vi "Indexing_Modbus.vi"(0 "Modbus master in":refnum<class "Modbus Master.lvclass">, 4 "Modbus Input":T1, 7 "error in (no error)":errorcluster) -> (20 "Modbus master out":refnum<class "Modbus Master.lvclass">, 27 "error out":errorcluster)   [LabVIEW 2021]
uses:
  <vilib>/Modbus/master/Modbus Master.lvclass
  Controls/Modbus Input.ctl
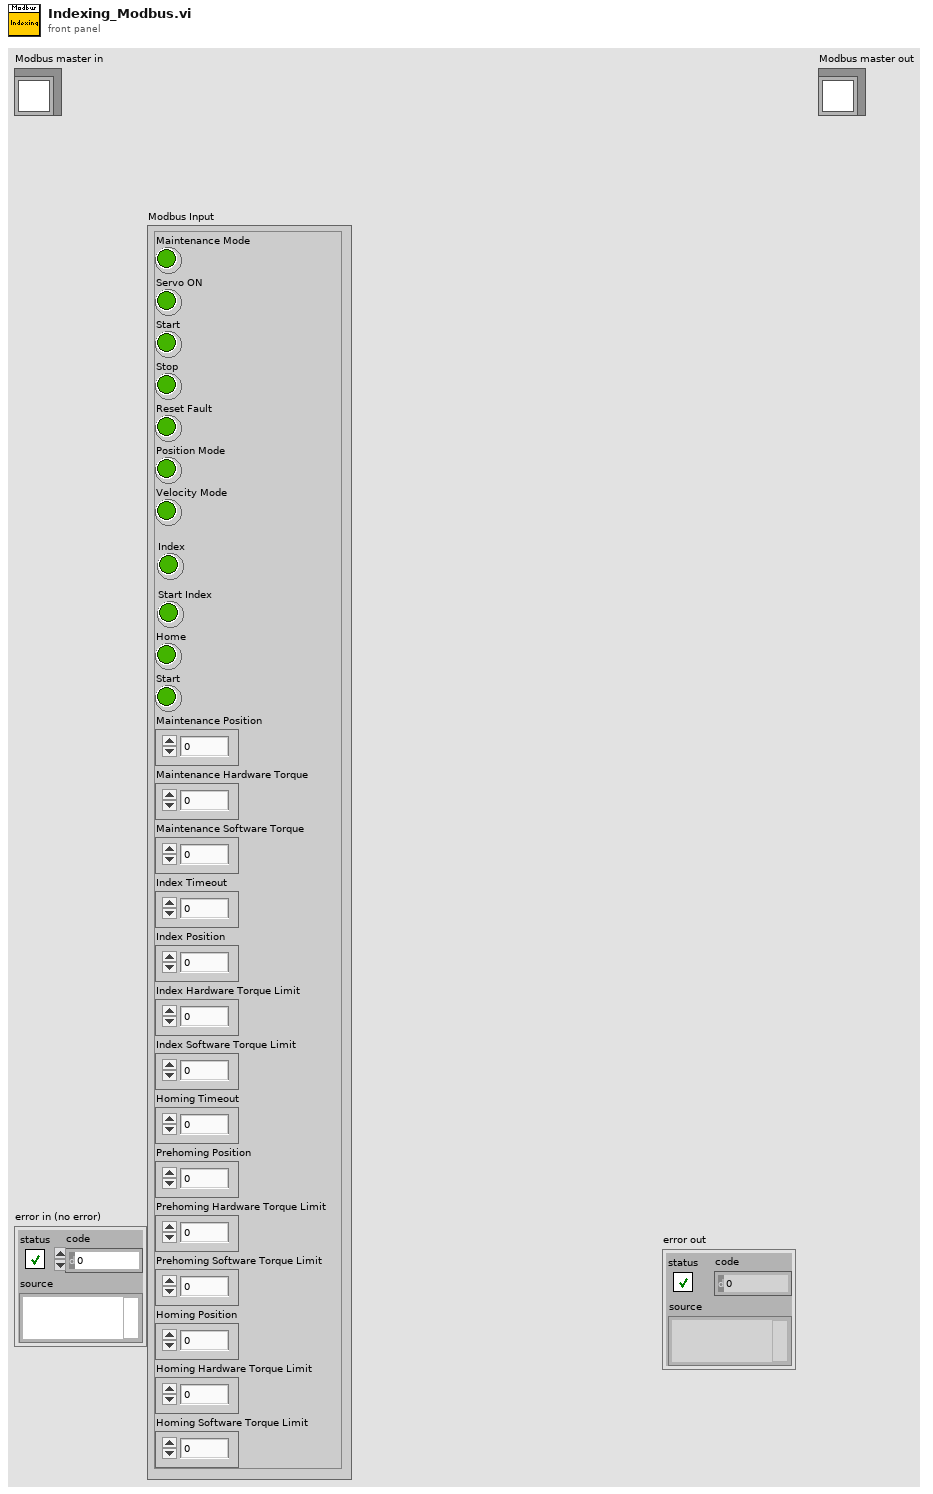
[diagram p1: front panel]
types:
  T1 = typedef "Modbus Input.ctl" = cluster{"Maintenance Mode":bool, "Servo ON":bool, "Start":bool, "Stop":bool, "Reset Fault":bool, "Position Mode":bool, "Velocity Mode":bool, "Index":bool, "Start Index":bool, "Home":bool, "Start":bool, "Maintenance Position":i32, "Maintenance Hardware Torque":u16, "Maintenance Software Torque":u16, "Index Timeout":i16, "Index Position":i32, "Index Hardware Torque Limit":u16, "Index Software Torque Limit":u16, "Homing Timeout":i16, "Prehoming Position":i32, "Prehoming Hardware Torque Limit":u16, "Prehoming Software Torque Limit":u16, "Homing Position":i32, "Homing Hardware Torque Limit":u16, "Homing Software Torque Limit":u16}
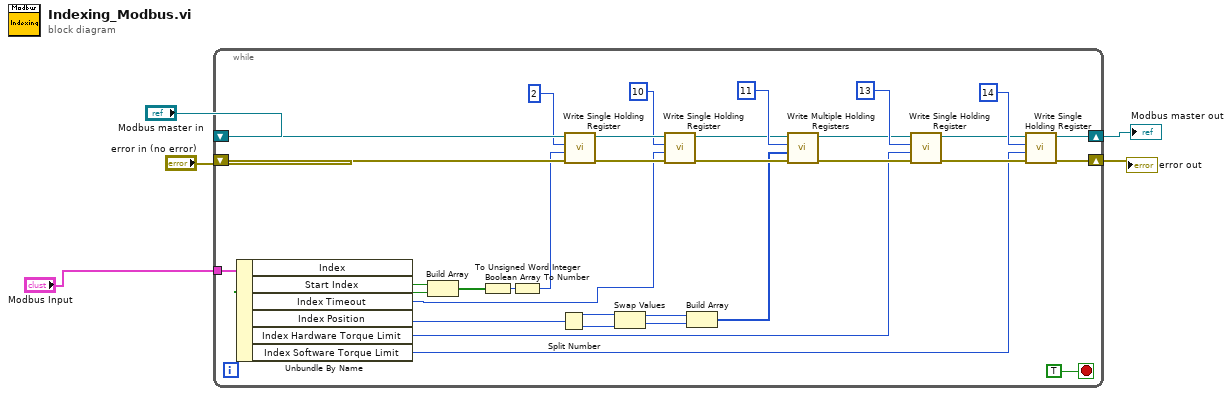
[diagram p0: block diagram]
diagram:
  n1 = while {
    shift-right: [w20] -> w3
    shift-left: "Modbus master in" -> [w38]
    shift-right: [w19] -> w2
    shift-left: "error in (no error)" -> [w37]
    tunnel: "Modbus Input" -> [w17]
    stop <- TRUE stop-if-true
    n2 = Unbundle By Name(w17) -> ("Index"=w16:bool, "Start Index"=w15:bool, "Index Timeout"=w14:i16, "Index Position"=w13:i32, "Index Hardware Torque Limit"=w7:u16, "Index Software Torque Limit"=w6:u16)
    n3 = Build Array(w16, w15) -> (w35:bool[])
    n4 = Boolean Array To Number(Boolean array=w35) -> (number=w34:u32)
    n5 = To Unsigned Word Integer(number=w34) -> (unsigned 16bit integer=w33:u16)
    n6 = Split Number(x=w13) -> (hi(x)=w12:u16, lo(x)=w11:u16)
    n7 = call-dynamic "Write Single Holding Register.vi"("error in (no error)"=w37, "holding register value"=w33, "address"=u16 2, "Modbus master in"=w38) -> ("error out"=w31:errorcluster, "Modbus master out"=w32:refnum<class "Modbus Master.lvclass">)  [unwired: 6 in]
    n8 = Swap Values(12:w12, 14:w11) -> (1:w10:u16, 3:w9:u16)  [unwired: 1 in]
    n9 = call-dynamic "Write Single Holding Register.vi"("error in (no error)"=w31, "holding register value"=w14, "address"=u16 10, "Modbus master in"=w32) -> ("error out"=w27:errorcluster, "Modbus master out"=w28:refnum<class "Modbus Master.lvclass">)  [unwired: 6 in]
    n10 = Build Array(w10, w9) -> (w8:u16[])
    n11 = call-dynamic "Write Multiple Holding Registers.vi"("error in (no error)"=w27, "holding register values"=w8, "starting address"=u16 11, "Modbus master in"=w28) -> ("error out"=w24:errorcluster, "Modbus master out"=w23:refnum<class "Modbus Master.lvclass">)  [unwired: 6 in]
    n12 = call-dynamic "Write Single Holding Register.vi"("error in (no error)"=w24, "holding register value"=w7, "address"=u16 13, "Modbus master in"=w23) -> ("error out"=w21:errorcluster, "Modbus master out"=w22:refnum<class "Modbus Master.lvclass">)  [unwired: 6 in]
    n13 = call-dynamic "Write Single Holding Register.vi"("error in (no error)"=w21, "holding register value"=w6, "address"=u16 14, "Modbus master in"=w22) -> ("error out"=w19:errorcluster, "Modbus master out"=w20:refnum<class "Modbus Master.lvclass">)  [unwired: 6 in]
  }
  "Modbus master out" <- w3
  "error out" <- w2
